vi "CMD_Run.vi"(1 "Line":string) -> (0 "Done":bool)   [LabVIEW 2015]
panel:
  in  "Parameters":i32[](array[numeric])=[1, 1, 1, 1]
  in  "Subcommands":string[](array[string])=["motor", "at", "for", "until"]
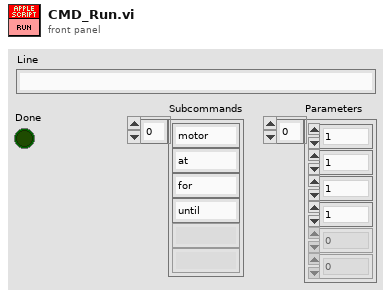
[diagram p1: front panel]
types:
  T1 = typedef "WPI_MotorControlDeviceRef.ctl" = cluster{"DeviceStatus":errorcluster, "Type":T2, "PWM":cluster{"PWM Channel":T3, "DeadBand":T4}, "CAN":cluster{"Device Number":u8, "Control Mode":T5, "Semaphore":T6, "Max Vout":dbl, "TalonSRX Control Mode":T7}, "Invert":bool}
  T2 = typedef "WPI_MotorControlType.ctl" = enum16{"PWM", "CAN", "CANTalonSRX"}
  T3 = typedef "FPGA_DIOPWMChannel.ctl" = enum8{"PWM 0", "PWM 1", "PWM 2", "PWM 3", "PWM 4", "PWM 5", "PWM 6", "PWM 7", "PWM 8", "PWM 9", "PWM MXP 0", "PWM MXP 1", "PWM MXP 2", "PWM MXP 3", "PWM MXP 4", "PWM MXP 5", "PWM MXP 6", "PWM MXP 7", "PWM MXP 8", "PWM MXP 9", "Invalid"}
  T4 = typedef "WPI_PWMDeadband.ctl" = cluster{"Name":string, "maxPositivePwm":i32, "minPositivePwm":i32, "centerPwm":i32, "maxNegativePwm":i32, "minNegativePwm":i32, "angularRange":u16}
  T5 = typedef "WPI_CANJaguar_ControlMode.ctl" = enum8{"Percent VBus", "Current", "Speed", "Position", "Voltage"}
  T6 = typedef "Semaphore RefNum" = refnum<k1>
  T7 = typedef "WPI_CANTalonSRX_APIControlMode.ctl" = enum8{"Percent VBus", "Speed", "Position", "Slave", "Unchanged / Invalid", "Voltage Compensation", "Current", "Motion Profile"}
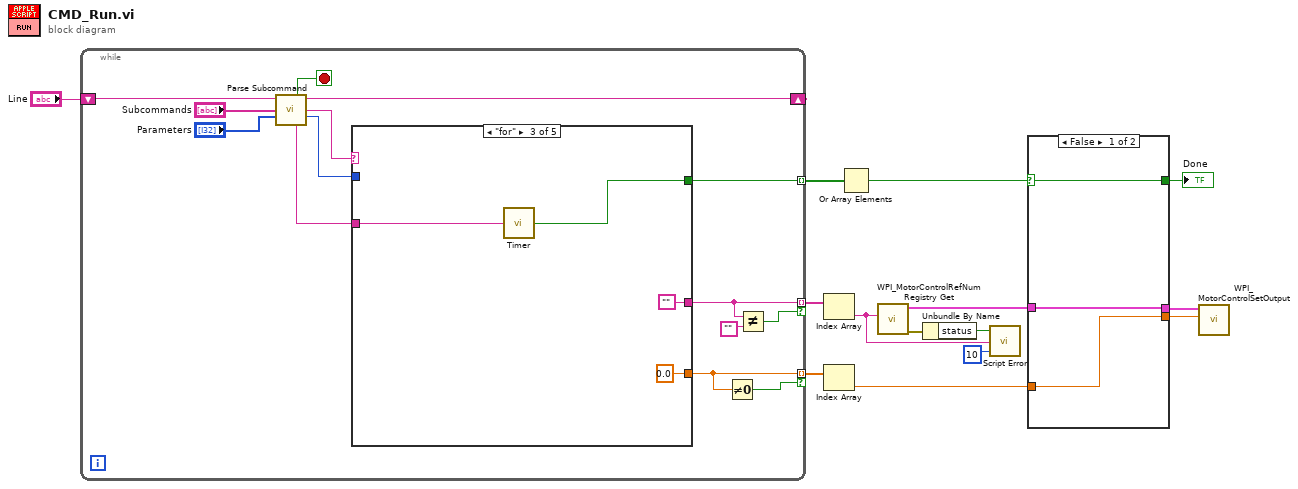
[diagram p0: block diagram]
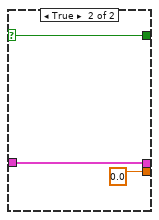
[diagram p2: hidden frame]
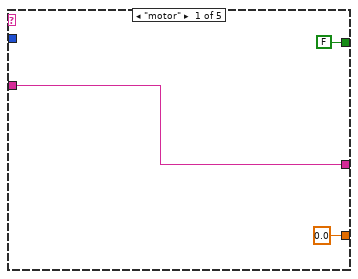
[diagram p3: hidden frame]
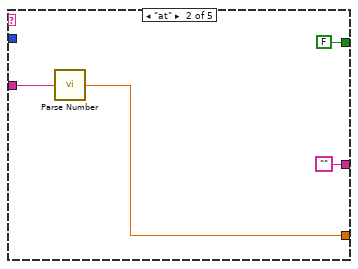
[diagram p4: hidden frame]
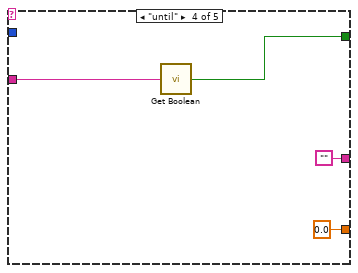
[diagram p5: hidden frame]
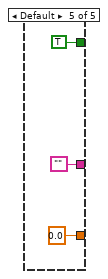
[diagram p6: hidden frame]
diagram:
  n1 = while {
    shift-right: [w25] -> _
    shift-left: "Line" -> [w28]
    tunnel: [w20] -> w13 mode=indexing
    tunnel: [w19] -> w12 mode=indexing if=w17
    tunnel: [w16] -> w11 mode=indexing if=w15
    stop <- w24 stop-if-true
    n2 = call "Parse Subcommand.vi"("Text In"=w28, "Subcommands"="Subcommands", "Parameters"="Parameters") -> ("Done"=w24:bool, "Text Out"=w25:string, "Subcommand"=w23:string, "# of Parameters"=w22:i32, "Parameter 1"=w21:string)  [unwired: 6 in, 2 out]
    n3 = case shown="\"for\"" w23 {
      tunnel: w22 -> [_ _ _ _ _]
      tunnel: w21 -> [w29 w35 w39 w43 _]
      tunnel: [FALSE FALSE ("Value") w36 w40 TRUE ("Value")] -> w20
      tunnel: [w29 "" "" "" ""] -> w19
      tunnel: [0.0 ("Number") w32 0.0 ("Number") 0.0 ("Number") 0.0 ("Number")] -> w16
      frame "motor" {
      }
      frame "at" {
        n4 = call "Parse Number.vi"("String"=w35) -> ("Number"=w32:dbl)
      }
      frame "for" {
        n5 = call "Timer.vi"("Seconds (string)"=w39) -> ("Done"=w36:bool)
      }
      frame "until" {
        n6 = call "Get Boolean.vi"("Name"=w43) -> ("Value"=w40:bool)
      }
      frame Default {
      }
    }
    n7 = Not Equal To 0?(x=w16) -> (x != 0?=w15:bool)
    n8 = Not Equal?(x=w19, y="") -> (x != y?=w17:bool)
  }
  n9 = Index Array(array=w12) -> (element=w1:string)  [unwired: 1 in]
  n10 = Index Array(array=w11) -> (element=w6:dbl)  [unwired: 1 in]
  n11 = Or Array Elements(Boolean array=w13) -> (logical OR=w10:bool)
  n12 = call <vilib>:"WPI_MotorControlRefNum Registry Get.vi"("refnum name"=w1) -> ("error out"=w4:errorcluster, "MotorControlDevRef"=w8:T1)  [unwired: 9 in]
  n13 = Unbundle By Name(w4) -> ("status"=w2:bool)
  n14 = call "Script Error.vi"("Error?"=w2, "Error Details"=w1, "Error Code"=10) -> ()  [unwired: 2 in, 1 out]
  n15 = case shown="False" w10 {
    selector: w10 -> [w49 w52]
    tunnel: [w49 w52] -> w9
    tunnel: w8 -> [w48 w51]
    tunnel: [w48 w51] -> w7
    tunnel: w6 -> [w47 _]
    tunnel: [w47 0.0] -> w5
    frame False {
    }
    frame True {
    }
  }
  "Done" <- w9
  n16 = call <vilib>:"WPI_MotorControlSetOutput.vi"("Output"=w5, "MotorControlDevRef"=w7) -> ()  [unwired: 7 in, 3 out]
